vi "evaluateVonKarman.vi"(9 "frequencies":dbl[](array[numeric]), 10 "lambda":dbl, 11 "vonKarmanFitEquation":string) -> (3 "Cluster":cluster{"frequencies":dbl[], "Y Values":dbl[]})   [LabVIEW 2013]
uses:
  <vilib>/gmath/NI_Gmath.lvlib
panel:
  out "result string":string
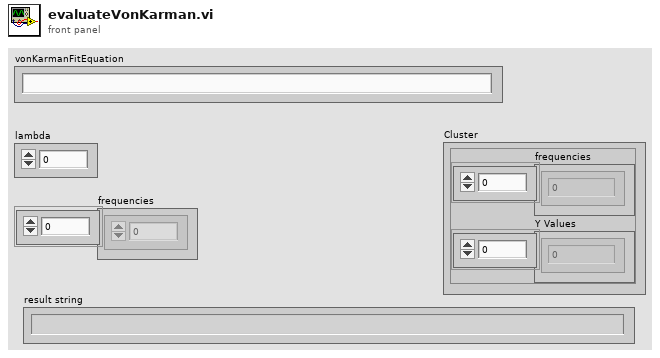
[diagram p1: front panel]
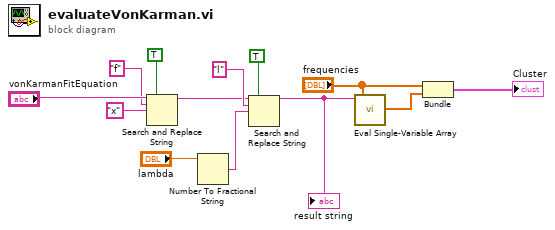
[diagram p0: block diagram]
diagram:
  n1 = Search and Replace String(replace all?=TRUE ("replace all? (F)"), input string="vonKarmanFitEquation", search string="f", replace string="x" ("replace string (\"\")")) -> (result string=w4:string)  [unwired: 4 in, 3 out]
  n2 = Number To Fractional String(number="lambda") -> (F-format string=w1:string)  [unwired: 3 in]
  n3 = Search and Replace String(replace all?=TRUE ("replace all? (F)"), input string=w4, search string="l", replace string=w1) -> (result string=w3:string)  [unwired: 4 in, 3 out]
  "result string" <- w3
  n4 = call <vilib>:"Eval Single-Variable Array.vi"("X Values"="frequencies", "formula"=w3) -> ("Y Values"=w11:dbl[])  [unwired: 1 in, 1 out]
  n5 = Bundle("frequencies"="frequencies", "Y Values"=w11) -> (→"Cluster":cluster{"frequencies":dbl[], "Y Values":dbl[]})  [unwired: 1 in]
